vi "Delete.vi"(5 "Delete all found":bool, 6 "$Path or Item Name":string, 7 "error in (no error)":errorcluster, 9 "Offset":i32, 10 "JSON":string="{}") -> (0 "error out":errorcluster, 1 "<JSON> First Deleted Item":string, 2 "Number Deleted":i32, 3 "<JSON>":string caption="<JSON>With Item Deleted")   [LabVIEW 2019, in "JSONtext.lvlib"]
doc: "Deletes JSON item at the JSON Path specified. If \"Delete all found\" is True, will delete all items matching the path. Else will just delete the first found."
uses:
  JSONtext.lvlib
  Parsing/Parsing State.ctl
  support/Quote and Escape JSON string.vi
  Parsing/Advance past Line Ending.vi
  support/quote and escape json string 2.vi
  Parsing/Parse Full Path or Item Name.vi
  Parsing/Path Notation End Name.vi
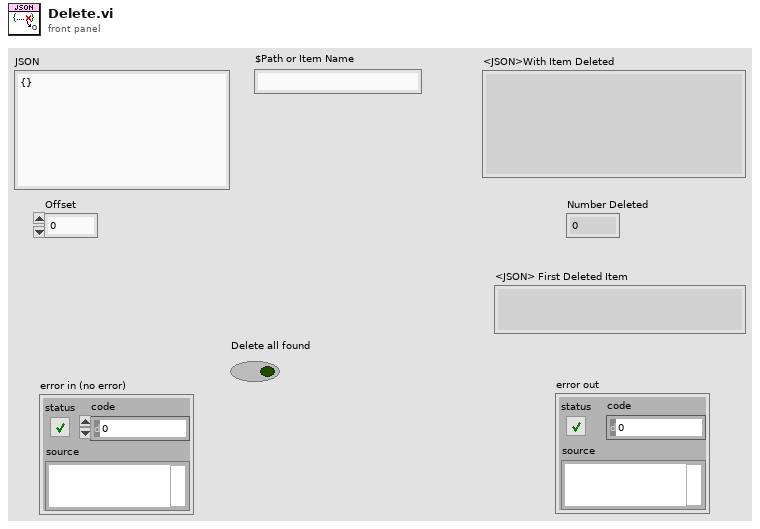
[diagram p1: front panel]
types:
  T1 = typedef "JSONtext.lvlib/Found Items.ctl" = cluster{"Item offset":i32, "Offset past Item":i32, "Name offset":i32, "Offset past Name":i32, "Found":bool, "Item Type":T2, "Item Index":i32, "Start Offset":i32, "Comma Needed For Insert":bool}
  T2 = typedef "JSONtext.lvlib/Parsing State.ctl" = enum16{"Parser Error", "Object", "Array", "String", "Number/Other", "Leading Whitespace", "Object end", "Array end", "Value end"}
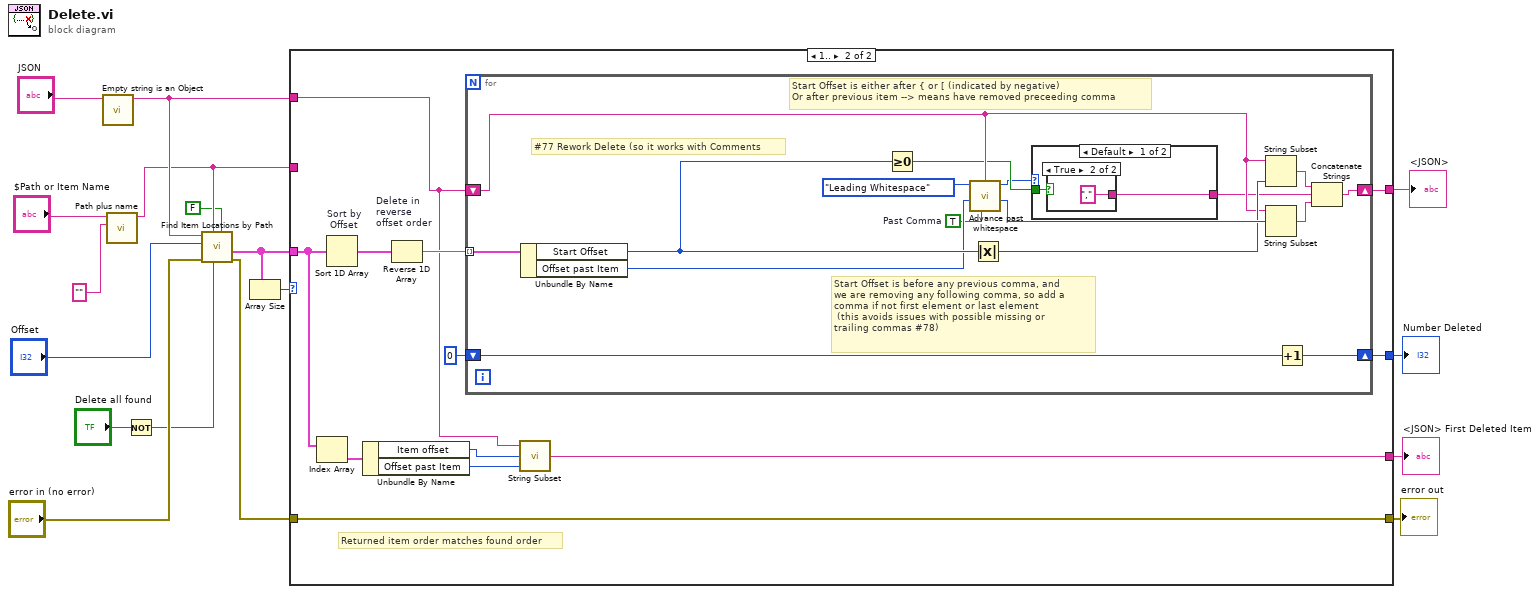
[diagram p0: block diagram]
diagram:
  n1 = call "Empty string is an Object.vi"("JSON Input"="JSON") -> ("<JSON>Object"=w12:string)  [unwired: 10 in]
  n2 = call "Path plus name.vi"("Item Name"="", "Object (or Item) Path"="$Path or Item Name") -> ("Relative Path or JSON-format name"=w9:string)  [unwired: 7 in, 2 out]
  n3 = Not(x="Delete all found") -> (.not. x?=w2:bool)
  n4 = call "Find Item Locations by Path.vi"("Insertion point if not found"=FALSE, "Only return first found"=w2, "Path"=w9, "error in (no error)"="error in (no error)", "Offset"="Offset", "JSON"=w12) -> ("error out"=w5:errorcluster, "Items"=w7:T1[])  [unwired: 4 in]
  n5 = Array Size(array=w7) -> (size(s)=w6:i32)
  n6 = case shown="1.." w6 {
    tunnel: [w19 w30] -> w17
    tunnel: w12 -> [w19 w21]
    tunnel: w7 -> [_ w23]
    tunnel: w5 -> [w18 w31]
    tunnel: w9 -> [_ _]
    tunnel: [w18 w31] -> w14
    tunnel: [_ w26] -> w3
    tunnel: [_ w20] -> w1
    frame 0, Default {
    }
    frame 1.. {
      # "Returned item order matches found order"
      n7 = Index Array(array=w23) -> (element=w22:T1)  [unwired: 1 in]
      n8 = Sort 1D Array "Sort by\n Offset"(array=w23) -> (sorted array=w28:T1[])
      n9 = Unbundle By Name(w22) -> ("Item offset"=w25:i32, "Offset past Item"=w24:i32)
      n10 = Reverse 1D Array "Delete in \nreverse\noffset order"(array=w28) -> (reversed array=w29:T1[])
      n11 = for {
        tunnel: w29 -> [w44] mode=indexing
        shift-right: [w46] -> w30
        shift-left: w21 -> [w43]
        shift-right: [w42] -> w26
        shift-left: 0 -> [w41]
        w34 = TRUE  # Past Comma
        # "Start Offset is either after { or [ (indicated by negative)\nOr after previous item --> means have removed preceeding comma"
        # "Start Offset is before any previous comma, and\nwe are removing any following comma, so add a \ncomma if not first element or last element\n (this avoids issues with possible missing or \ntrailing commas #78)"
        # "#77 Rework Delete (so it works with Comments"
        n12 = Unbundle By Name(w44) -> ("Start Offset"=w38:i32, "Offset past Item"=w37:i32)
        n13 = Greater Or Equal To 0?(x=w38) -> (x >= 0?=w33:bool)
        n14 = call "Advance past whitespace.vi"("Past Comma"=w34, "JSON"=w43, "Offset"=w37, "Parser State in"=Parsing_State."Leading Whitespace" ("State")) -> ("Offset of first non-whitespace"=w47:i32, "Parser State"=w32:T2)  [unwired: 5 in, 1 out]
        n15 = Absolute Value(x=w38) -> (abs(x)=w45:i32)
        n16 = case shown="Default" w32 {
          tunnel: [w49 _] -> w36
          tunnel: w33 -> [w48 _]
          frame Default {
            n17 = case shown="True" w48 {
              tunnel: [_ ","] -> w49
              frame False {
              }
              frame True {
              }
            }
          }
          frame "Object end", "Array end" {
          }
        }
        n18 = String Subset(string=w43, length (rest)=w45) -> (substring=w40:string)  [unwired: 1 in]
        n19 = String Subset(string=w43, offset (0)=w47) -> (substring=w39:string)  [unwired: 1 in]
        n20 = Increment(x=w41) -> (x+1=w42:i32)
        n21 = Concatenate Strings(w40, w36, w39) -> (w46:string)
      }
      n22 = call "String Subset.vi"("Offset past End"=w24, "Start offset"=w25, "JSON"=w21) -> ("substring"=w20:string)  [unwired: 2 in]
    }
  }
  "<JSON>" <- w17
  "error out" <- w14
  "Number Deleted" <- w3
  "<JSON> First Deleted Item" <- w1
